vi "PC_Handshake.vi"(0 "VISA resource name":refnum<visa-resource-name>="COM6", 1 "error in":errorcluster) -> (2 "VISA resource name out":refnum<visa-resource-name>, 3 "error out":errorcluster, 4 "Handshake Successful?":bool)   [LabVIEW 2014]
panel:
  out "String from \nmyRIO":string
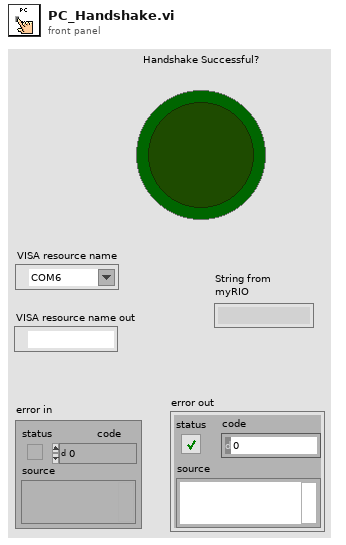
[diagram p1: front panel]
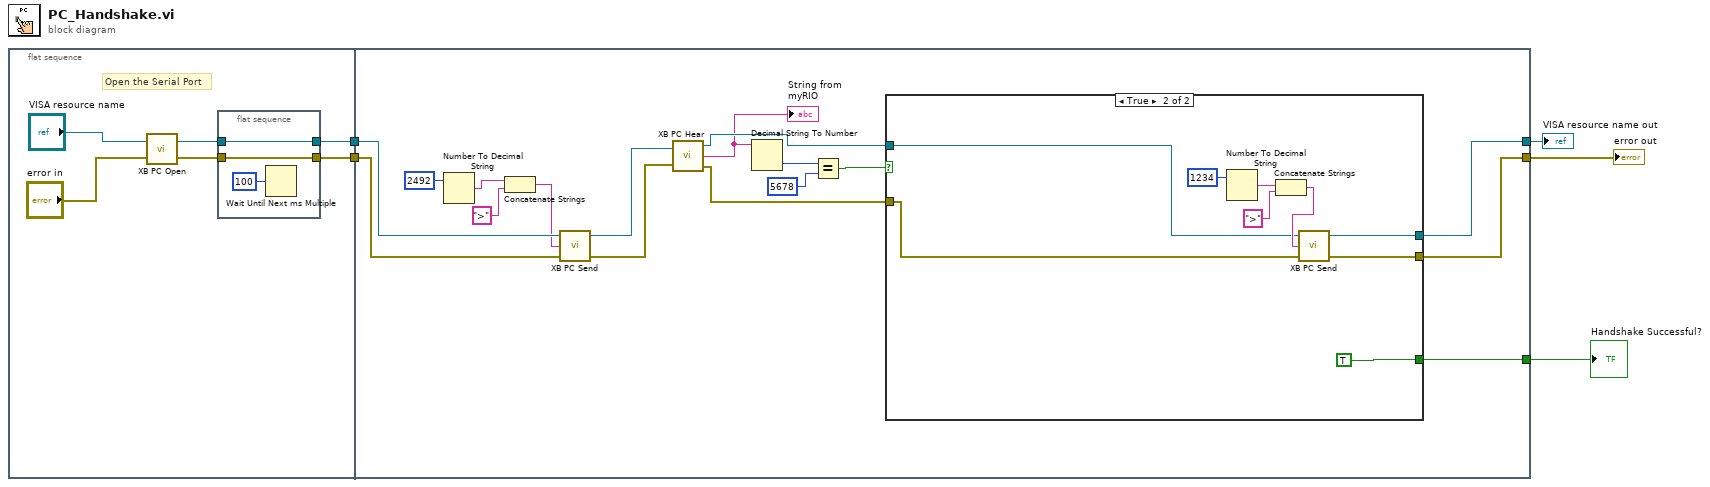
[diagram p0: block diagram]
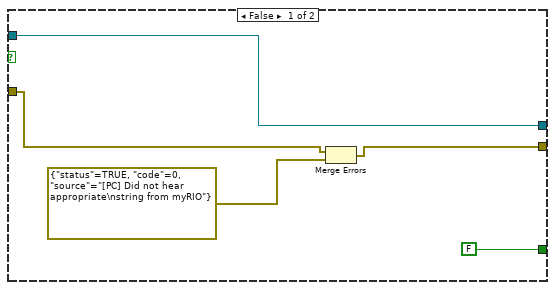
[diagram p2: hidden frame]
diagram:
  n1 = flat-sequence {
    tunnel: [w7] -> w5
    tunnel: [w6] -> w4
    tunnel: [w28] -> w2
    tunnel: [w29] -> w1
    tunnel: w5 -> [w31]
    tunnel: w4 -> [w30]
    tunnel: [w27] -> w3
    frame #0 {
      # "Open the Serial Port"
      n2 = call "XB PC Open.vi"("error in (no error)"="error in", "VISA resource name"="VISA resource name") -> ("error out"=w10:errorcluster, "VISA resource name out"=w11:refnum<visa-resource-name>)
      n3 = flat-sequence {
        tunnel: w11 -> [w12]
        tunnel: w10 -> [w13]
        tunnel: [w13] -> w6
        tunnel: [w12] -> w7
        frame #0 {
          n4 = Wait Until Next ms Multiple(millisecond multiple=u32 100) -> ()  [unwired: 1 out]
        }
      }
    }
    frame #1 {
      n5 = Number To Decimal String(number=2492) -> (decimal integer string=w23:string)  [unwired: 1 in]
      n6 = Concatenate Strings(w23, ">" ("string")) -> (w21:string)
      n7 = call "XB PC Send.vi"("error in (no error)"=w30, "String"=w21, "VISA resource name"=w31) -> ("error out"=w24:errorcluster, "VISA resource name out"=w25:refnum<visa-resource-name>)  [unwired: 1 out]
      n8 = call "XB PC Hear.vi"("VISA resource name"=w25, "error in (no error)"=w24) -> ("VISA resource name out"=w17:refnum<visa-resource-name>, "String Received"=w15:string, "error out"=w18:errorcluster)
      "String from \nmyRIO" <- w15
      n9 = Decimal String To Number(string=w15) -> (number=w20:i32)  [unwired: 2 in, 1 out]
      n10 = Equal?(x=w20, y=5678) -> (x = y?=w16:bool)
      n11 = case shown="True" w16 {
        tunnel: [w36 w45] -> w29
        tunnel: [w33 w44] -> w28
        tunnel: w18 -> [w35 w38]
        tunnel: w17 -> [w36 w39]
        tunnel: [FALSE TRUE] -> w27
        frame False {
          n12 = Merge Errors(w35, errorcluster {"status"=TRUE, "code"=0, "source"="[PC] Did not hear appropriate\nstring from myRIO"} ("error out")) -> (w33:errorcluster)
        }
        frame True {
          n13 = Number To Decimal String(number=1234) -> (decimal integer string=w41:string)  [unwired: 1 in]
          n14 = Concatenate Strings(w41, ">" ("string")) -> (w40:string)
          n15 = call "XB PC Send.vi"("error in (no error)"=w38, "String"=w40, "VISA resource name"=w39) -> ("error out"=w44:errorcluster, "VISA resource name out"=w45:refnum<visa-resource-name>)  [unwired: 1 out]
        }
      }
    }
  }
  "Handshake Successful?" <- w3
  "error out" <- w2
  "VISA resource name out" <- w1
